vi "RX-SIM-SIS-UDP.vi"() -> ()   [LabVIEW 2018]
uses:
  <vilib>/Platform/TimedLoop/XDataNode/timing_clust.ctl
  <vilib>/Platform/TimedLoop/XDataNode/nitl_modes.ctl
  <vilib>/Platform/TimedLoop/XDataNode/wakeup.ctl
  Global Variables.vi
  <vilib>/Platform/TimedLoop/XDataNode/XDataNode.xnode
  <vilib>/Platform/TimedLoop/XDataNode/XDNodeRunTimeDep.lvlib
panel:
  in  "Stop":bool
  out "SIM-SIS-RX-ARRAY":dbl[](array[numeric])
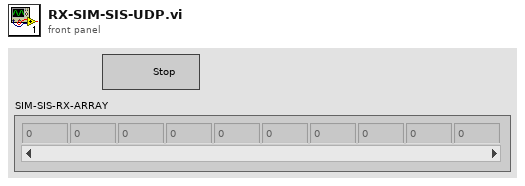
[diagram p1: front panel]
types:
  T1 = typedef "XDNodeRunTimeDep.lvlib/timing_clust.ctl" = cluster{"Expected End [f-1]":u64, "Actual End [f-1]":u64, "Finished Late? [f-1]":bool, "Expected End [i-1]":u64, "Actual End [i-1]":u64, "Finished Late? [i-1]":bool, "Expected Start [i]":u64, "Actual Start [i]":u64, "Expected Start [f]":u64, "Actual Start [f]":u64, "Source Name":string, "Structure Name":string, "Period":i64, "Deadline":i64, "Offset":i64, "Start":i64, "Priority":i32, "Timeout":i32, "Mode":T2, "Wakeup Reason":T3, "Error":errorcluster, "Source Type":string, "Secondary Source Type":string, "Global End Time":u64, "Global Start Time":u64, "Frame Duration":u64, "Iteration Duration":u64, "Assigned CPU":i32, "I/O Scan Engine Mode":u32}
  T2 = typedef "XDNodeRunTimeDep.lvlib/nitl_modes.ctl" = enum32{"No Change", "Process missed periods, maintain original phase", "Discard missed periods, maintain original phase", "Process missed periods, ignore original phase", "Discard missed periods, ignore original phase"}
  T3 = typedef "XDNodeRunTimeDep.lvlib/wakeup.ctl" = enum32{"Normal", "Aborted", "Asynchronous wakeup", "Timing source error", "Timed loop error", "Timeout"}
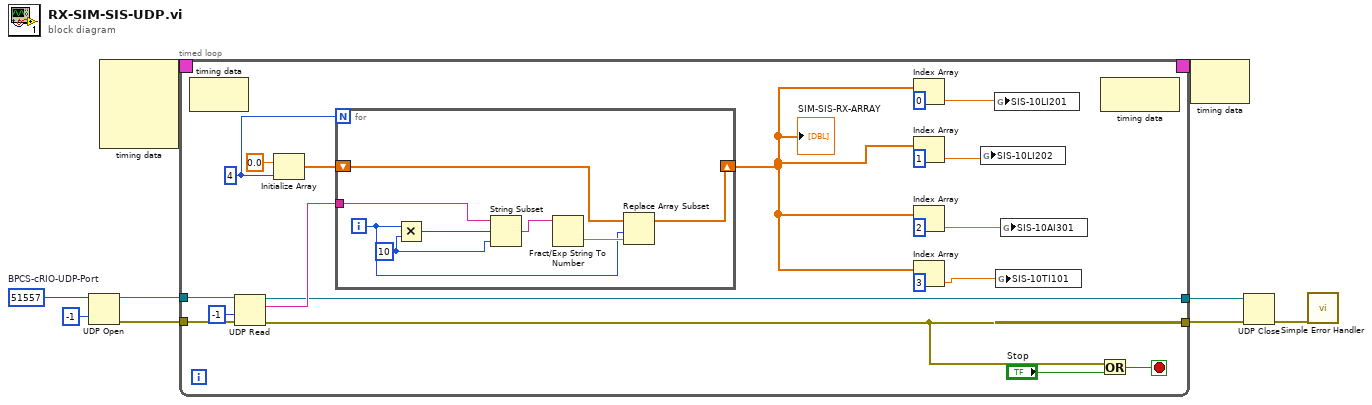
[diagram p0: block diagram]
diagram:
  w7 = u16 51557  # BPCS-cRIO-UDP-Port
  n1 = UDP Open(9:-1 ("timeout ms (25000)"), 11:w7) -> (port=w6:refnum<k16>, 0:w5:errorcluster)  [unwired: 3 in, 1 out]
  n2 = node-c288() -> (w9:T1)  [unwired: 4 in]
  n3 = timed-loop {
    timing: w9 -> [_]
    timing-out: [_] -> w8
    tunnel: w6 -> [w27]
    tunnel: w5 -> [w26]
    tunnel: [w24] -> w3
    tunnel: [w23] -> w2
    stop <- w28 stop-if-true
    w20 = 4 ("dimension size")
    n4 = node-c288() -> ()  [unwired: 1 in, 1 out]
    n5 = UDP Read(connection ID=w27, timeout ms (25000)=-1, 8:w26) -> (data out=w25:string, error out=w23:errorcluster, 3:w24:refnum<k16>)  [unwired: 3 out]
    n6 = Initialize Array(0.0 ("element"), w20) -> (w21:dbl[])
    n7 = for {
      N: w20 -> [_]
      tunnel: w25 -> [w36]
      shift-right: [w32] -> w15
      shift-left: w21 -> [w31]
      i -> [w33]
      w30 = 10 ("y")
      n8 = Multiply(x=w33, y=w30) -> (x*y=w35:i32)
      n9 = String Subset(string=w36, offset (0)=w35, length (rest)=w30) -> (substring=w37:string)
      n10 = Fract/Exp String To Number(string=w37) -> (number=w34:dbl)  [unwired: 3 in, 1 out]
      n11 = Replace Array Subset(array=w31, new element=w34, index=w33) -> (w32:dbl[])
    }
    "SIM-SIS-RX-ARRAY" <- w15
    n12 = Index Array(array=w15, index=0) -> (element=w13:dbl)
    n13 = Index Array(array=w15, index=1) -> (element=w12:dbl)
    n14 = Index Array(array=w15, index=2) -> (element=w11:dbl)
    n15 = Index Array(array=w15, index=3) -> (element=w10:dbl)
    n16 = global write "Global Variables.vi" "SIS-10LI202"(w12) -> ()
    n17 = global write "Global Variables.vi" "SIS-10LI201"(w13) -> ()
    n18 = global write "Global Variables.vi" "SIS-10TI101"(w10) -> ()
    n19 = global write "Global Variables.vi" "SIS-10AI301"(w11) -> ()
    n20 = Or(x=w23, y="Stop") -> (x .or. y?=w28:bool)
    n21 = node-c288() -> ()  [unwired: 1 in, 1 out]
  }
  n22 = node-c288(w8) -> ()  [unwired: 1 out]
  n23 = UDP Close(connection ID=w3, 8:w2) -> (error out=w4:errorcluster)  [unwired: 1 out]
  n24 = call <vilib>:"Simple Error Handler.vi"("error in (no error)"=w4) -> ()  [unwired: 4 in, 5 out]
